vi "SVD Decomposition.vi"   [LabVIEW 2010, in "NI_AALPro.lvlib"]
doc: "Computes the singular value decomposition (SVD) of the m x n matrix <B>A</B>. Wire data to the <B>A</B> input to determine the polymorphic instance to use or manually select the instance."
uses:
  NI_AALPro.lvlib
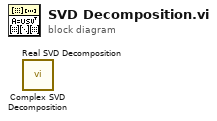
[diagram p0: block diagram]
diagram:
  n1 = call "Complex SVD Decomposition.vi"() -> ()  [unwired: 7 in, 5 out]
  n2 = call "Real SVD Decomposition.vi"() -> ()  [unwired: 7 in, 5 out]
